vi "Create Notifiers.vi"(8 "error in":errorcluster) -> (0 "error out":errorcluster, 3 "Notifiers":T1)   [LabVIEW 2022 SP3]
uses:
  Notifiers.ctl
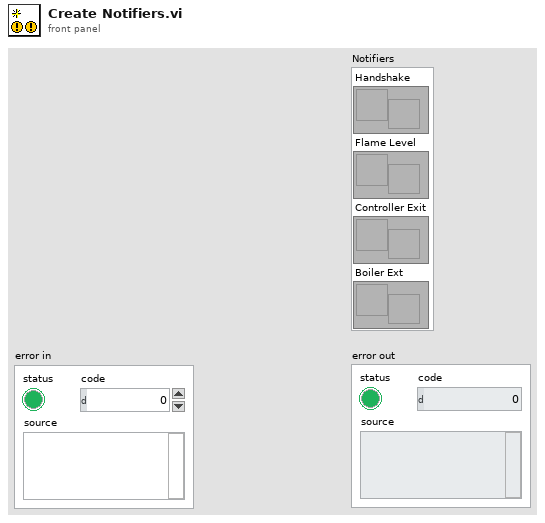
[diagram p1: front panel]
types:
  T1 = typedef "Notifiers.ctl" = cluster{"Handshake":refnum<notifier>, "Flame Level":refnum<notifier>, "Controller Exit":refnum<notifier>, "Boiler Ext":refnum<notifier>}
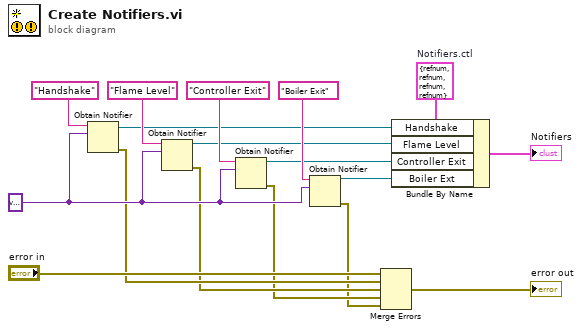
[diagram p0: block diagram]
diagram:
  w11 = T1 {"Handshake"=refnum, "Flame Level"=refnum, "Controller Exit"=refnum, "Boiler Ext"=refnum}  # Notifiers.ctl
  w13 = variant
  n1 = Obtain Notifier(name (unnamed)="Handshake", notification data type=w13) -> (notifier out=w12:refnum<notifier>, error out=w5:errorcluster)  [unwired: 2 in, 1 out]
  n2 = Obtain Notifier(name (unnamed)="Flame Level", notification data type=w13) -> (notifier out=w10:refnum<notifier>, error out=w4:errorcluster)  [unwired: 2 in, 1 out]
  n3 = Obtain Notifier(name (unnamed)="Controller Exit", notification data type=w13) -> (notifier out=w9:refnum<notifier>, error out=w3:errorcluster)  [unwired: 2 in, 1 out]
  n4 = Obtain Notifier(name (unnamed)="Boiler Exit", notification data type=w13) -> (notifier out=w8:refnum<notifier>, error out=w2:errorcluster)  [unwired: 2 in, 1 out]
  n5 = Merge Errors("error in", w5, w4, w3, w2) -> (→"error out":errorcluster)
  n6 = Bundle By Name(cluster=w11, "Handshake"=w12, "Flame Level"=w10, "Controller Exit"=w9, "Boiler Ext"=w8) -> (→"Notifiers":T1)
